vi "Result string to Boolean.vi"(11 "Result String":string) -> (3 "Boolean":bool)   [LabVIEW 2021]
doc: "string :1 ,OK ,True, disable to True; other string to false"
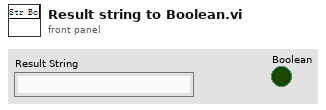
[diagram p1: front panel]
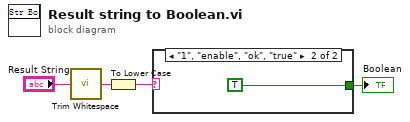
[diagram p0: block diagram]
diagram:
  n1 = call <vilib>:"Trim Whitespace.vi"("string"="Result String") -> ("trimmed string"=w1:string)  [unwired: 1 in]
  n2 = To Lower Case(string=w1) -> (all lower case string=w4:string)
  n3 = case shown="\"1\", \"enable\", \"ok\", \"true\"" w4 {
    tunnel: [_ TRUE] -> w2
    frame "False", Default {
    }
    frame "1", "enable", "ok", "true" {
    }
  }
  "Boolean" <- w2
